vi "Configure Inheritance.vi"(8 "error in (no error)":errorcluster, 11 "Process Generator in":refnum<class "Process Generator.lvclass">) -> (0 "error out":errorcluster, 3 "Process Generator out":refnum<class "Process Generator.lvclass">)   [LabVIEW 2020, in "Process Generation.lvlib" / "Process Generator.lvclass"]
uses:
  Process Generator.lvclass
  Process Generator.lvclass/Process Generator.ctl
  Framework/Process/Process.lvclass
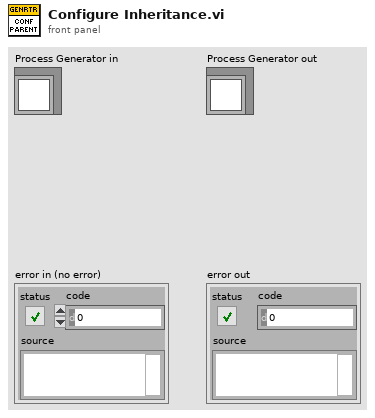
[diagram p1: front panel]
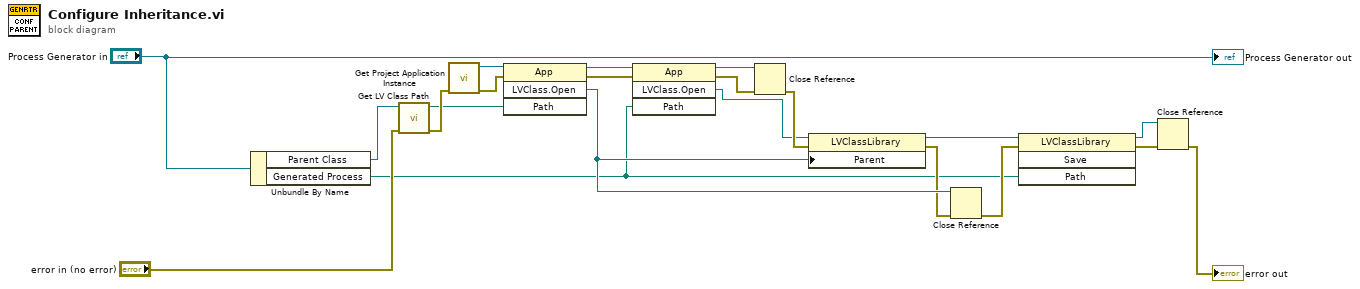
[diagram p0: block diagram]
diagram:
  n1 = Unbundle By Name("Process Generator in") -> ("Parent Class"=w21:refnum<class "Process.lvclass">, "Generated Process"=w4:path)
  n2 = call <vilib>:"Get LV Class Path.vi"("error in (no error)"="error in (no error)", "object"=w21) -> ("error out"=w17:errorcluster, "class path"=w9:path)  [unwired: 8 in]
  n3 = call "Get Project Application Instance.vi"("error in (no error)"=w17) -> ("error out"=w18:errorcluster, "Application out"=w16:refnum<vi>)  [unwired: 9 in]
  n4 = invoke class="App" method="LVClass.Open"(reference=w16, error in=w18, "Path"=w9) -> (reference out=w8:refnum<vi>, error out=w7:errorcluster, "LVClass.Open"=w14:refnum<vi>)  [unwired: 1 in, 1 out]
  n5 = invoke class="App" method="LVClass.Open"(reference=w8, error in=w7, "Path"=w4) -> (reference out=w6:refnum<vi>, error out=w5:errorcluster, "LVClass.Open"=w3:refnum<vi>)  [unwired: 1 in, 1 out]
  n6 = Close Reference(reference=w6, error in (no error)=w5) -> (error out=w19:errorcluster)
  n7 = property class="LVClassLibrary"(reference=w3, error in=w19, "Parent"=w14) -> (reference out=w10:refnum<vi>, error out=w11:errorcluster)
  n8 = Close Reference(reference=w14, error in (no error)=w11) -> (error out=w13:errorcluster)
  n9 = invoke class="LVClassLibrary" method="Save"(reference=w10, error in=w13, "Path"=w4) -> (reference out=w1:refnum<vi>, error out=w12:errorcluster)  [unwired: 1 in, 2 out]
  n10 = Close Reference(reference=w1, error in (no error)=w12) -> (error out=→"error out":errorcluster)
  "Process Generator out" <- "Process Generator in"
